vi "find_SpecObject_by_Name.vi"(10 "Spec Name":string, 11 "SpecObjects in":refnum<class "Spectrometer.lvclass">[](array[class])) -> (0 "index of found":i32, 1 "found InstrObject":refnum<class "instrument.lvclass">, 2 "found SpecObject":refnum<class "Spectrometer.lvclass">, 3 "SpecObjects out":refnum<class "Spectrometer.lvclass">[](array[class]))   [LabVIEW 2013]
doc: "Find the correct SpecObject by the Name of the Instrument"
uses:
  Classes/Spectrometer/Spectrometer.lvclass
  Classes/Instrument/instrument.lvclass
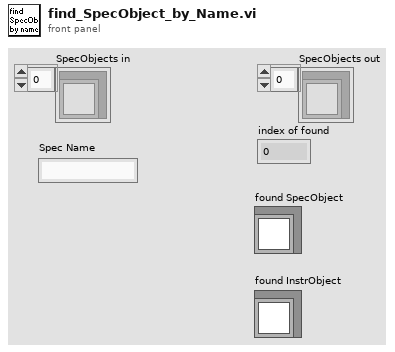
[diagram p1: front panel]
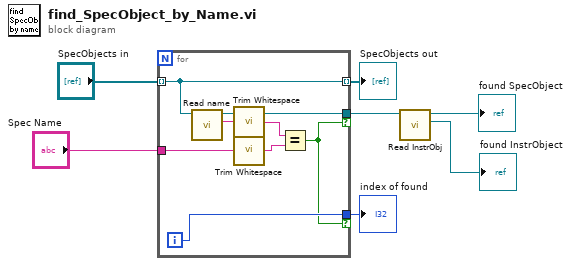
[diagram p0: block diagram]
diagram:
  n1 = for {
    tunnel: "SpecObjects in" -> [w10] mode=indexing
    tunnel: "Spec Name" -> [w14]
    tunnel: [w11] -> w6 if=w8
    tunnel: [w10] -> w2 mode=indexing
    tunnel: [w9] -> w1 if=w8
    i -> [w9]
    n2 = call-dynamic "Read name.vi"("Spectrometer in"=w10) -> ("name"=w15:string, "Spectrometer out"=w11:refnum<class "Spectrometer.lvclass">)  [unwired: 8 in, 1 out]
    n3 = call <vilib>:"Trim Whitespace.vi"("string"=w15) -> ("trimmed string"=w13:string)  [unwired: 1 in]
    n4 = call <vilib>:"Trim Whitespace.vi"("string"=w14) -> ("trimmed string"=w12:string)  [unwired: 1 in]
    n5 = Equal?(x=w13, y=w12) -> (x = y?=w8:bool)
  }
  "SpecObjects out" <- w2
  "index of found" <- w1
  n6 = call-dynamic "Read InstrObj.vi"("Spectrometer in"=w6) -> ("instrument.lvclass"=→"found InstrObject":refnum<class "instrument.lvclass">, "Spectrometer out"=→"found SpecObject":refnum<class "Spectrometer.lvclass">)  [unwired: 8 in, 1 out]
